vi "Get SpeedLimit(KB_s).vi"(8 "error in (no error)":errorcluster, 11 "FileTransferOptions in":refnum<class "FileTransferOptions.lvclass">) -> (0 "error out":errorcluster, 2 "SpeedLimit(KB/s)":i32, 3 "FileTransferOptions out":refnum<class "FileTransferOptions.lvclass">)   [LabVIEW 2015, in "WinSCP.lvlib" / "FileTransferOptions.lvclass"]
uses:
  FileTransferOptions.lvclass
  FileTransferOptions.lvclass/FileTransferOptions.ctl
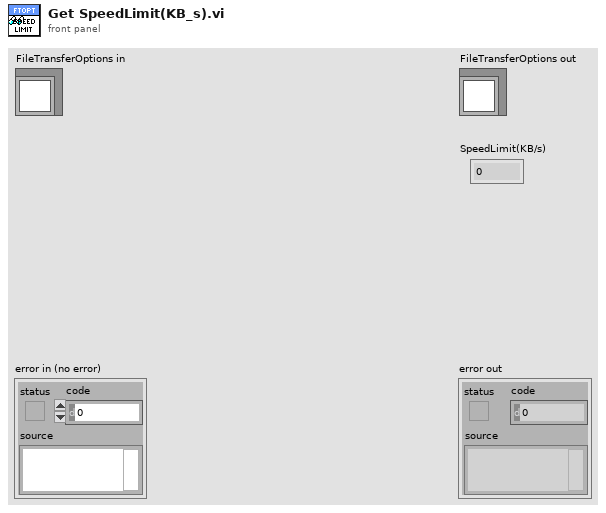
[diagram p1: front panel]
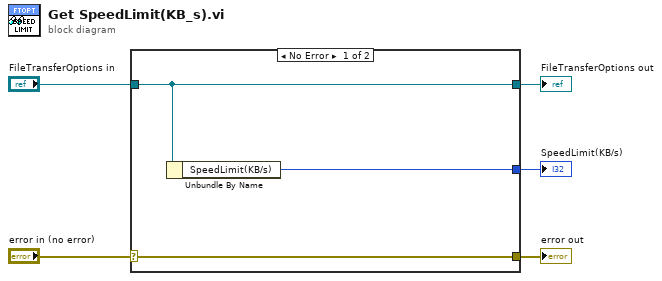
[diagram p0: block diagram]
diagram:
  n1 = case shown="No Error" "error in (no error)" {
    selector: "error in (no error)" -> [w8 w9]
    tunnel: [w8 w9] -> w4
    tunnel: [w7 w10] -> w2
    tunnel: "FileTransferOptions in" -> [w7 w10]
    tunnel: [w6 _] -> w1
    frame No Error {
      n2 = Unbundle By Name(w7) -> ("SpeedLimit(KB/s)"=w6:i32)
    }
    frame Error {
    }
  }
  "error out" <- w4
  "FileTransferOptions out" <- w2
  "SpeedLimit(KB/s)" <- w1
